vi "UpdateScanPan.vi"(4 "MainProgQEvent":refnum<user-event>, 6 "MainProgQ":refnum<queue>, 8 "error in (no error)":errorcluster caption="entrée d'erreur (pas d'erreur)", 10 "Function":i32, 11 "Experiment en entrée":refnum<class "Experiment.lvclass"> caption="DNL_LabVIEW Object in") -> (0 "error out":errorcluster caption="sortie d'erreur", 1 "NextPanPos":u32, 2 "PanScanFunc":string[](array[string]), 3 "Experiment en sortie":refnum<class "Experiment.lvclass"> caption="DNL_LabVIEW Object out")   [LabVIEW 2019, in "Experiment.lvclass"]
uses:
  Experiment.lvclass
  Experiment.lvclass/Experiment.ctl
  DevicesClass/BaseDevice/BaseDevice.lvclass
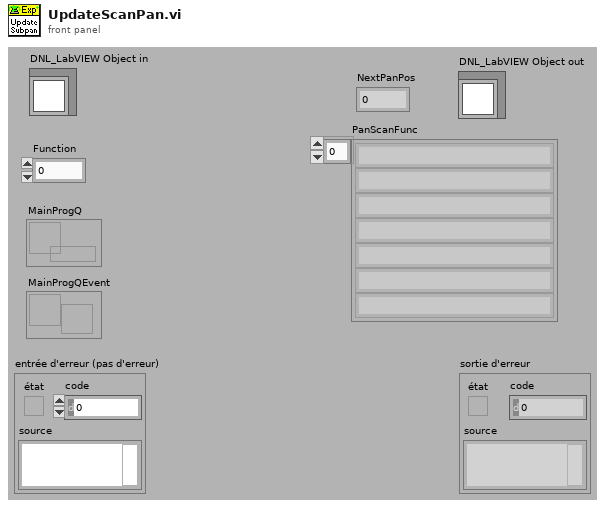
[diagram p1: front panel]
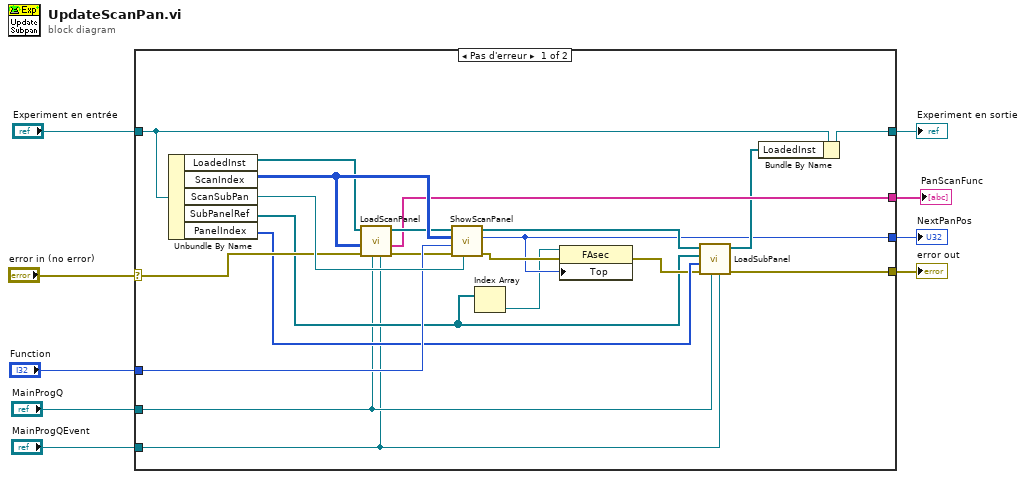
[diagram p0: block diagram]
diagram:
  n1 = case shown="Pas d'erreur" "error in (no error)" {
    selector: "error in (no error)" -> [w19 w32]
    tunnel: [w20 w32] -> w8
    tunnel: [w27 w31] -> w6
    tunnel: "Experiment en entrée" -> [w30 w31]
    tunnel: "Function" -> [w28 _]
    tunnel: [w23 _] -> w4
    tunnel: [w14 _] -> w3
    tunnel: "MainProgQ" -> [w11 _]
    tunnel: "MainProgQEvent" -> [w10 _]
    frame No Error {
      n2 = Unbundle By Name(w30) -> ("LoadedInst"=w18:refnum<class "BaseDevice.lvclass">[], "ScanIndex"=w26:i32[][], "ScanSubPan"=w29:refnum<vi>, "SubPanelRef"=w13:refnum<vi>[], "PanelIndex"=w17:i32[])
      n3 = call "LoadScanPanel.vi"("MainProgQEvent"=w10, "MainProgQ"=w11, "error in (no error)"=w19, "ScanIndex"=w26, "LoadedInst"=w18) -> ("sortie d'erreur"=w24:errorcluster, "PanScanFunc"=w23:string[], "LoadedInst Out"=w25:refnum<class "BaseDevice.lvclass">[])  [unwired: 3 in, 1 out]
      n4 = call "ShowScanPanel.vi"("SubPanel"=w29, "error in (no error)"=w24, "Function"=w28, "ScanIndex"=w26, "LoadedInst"=w25) -> ("sortie d'erreur"=w16:errorcluster, "NextPanPos"=w14:u32, "LoadedInst Out"=w22:refnum<class "BaseDevice.lvclass">[])  [unwired: 4 in]
      n5 = Index Array(array=w13) -> (element=w12:refnum<vi>)  [unwired: 1 in]
      n6 = property class="FAsec"(reference=w12, error in=w16, "Top"=w14) -> (error out=w15:errorcluster)  [unwired: 1 out]
      n7 = call "LoadSubPanel.vi"("MainProgQEvent"=w10, "MainProgQ"=w11, "error in (no error)"=w15, "PanelIndex"=w17, "SubPanel Refs"=w13, "LoadedInst"=w22) -> ("sortie d'erreur"=w20:errorcluster, "LoadedInst Out"=w21:refnum<class "BaseDevice.lvclass">[])  [unwired: 4 in]
      n8 = Bundle By Name(cluster=w30, "LoadedInst"=w21) -> (w27:refnum<class "Experiment.lvclass">)
    }
    frame Error {
    }
  }
  "error out" <- w8
  "Experiment en sortie" <- w6
  "PanScanFunc" <- w4
  "NextPanPos" <- w3
